vi "20 Log To File.vi"() -> ()   [LabVIEW 2014]
uses:
  <userlib>/_OpenG.lib/file/file.llb/Build Path - Traditional__ogtk.vi
  <vilib>/NI/LogRotate/LogRotate.lvclass
  Sensor Reading.ctl
  <vilib>/NI/LogRotate/options.ctl
panel:
  in  "Options":T1={"max file size (bytes)"=25000, "rotate count"=5, "max age (days)"=-1.0, "No archive dir"=TRUE, "Archive dir"=path ""}
  in  "Database File":path=path "C:/developer/New Model/database.txt"
  in  "Message Q":refnum<queue>
  in  "Data Q":refnum<queue>
  in  "Sensor Reading":T2
  # "INPUT PARAMETERS"
  # "INTERNAL VARIABLES - could possibly be set programatically..."
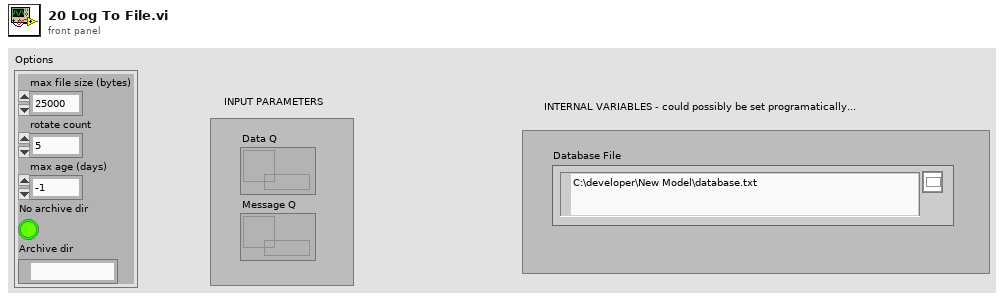
[diagram p1: front panel]
types:
  T1 = typedef "LogRotate.lvclass/options.ctl" = cluster{"max file size (bytes)":i64, "rotate count":u32, "max age (days)":dbl, "No archive dir":bool, "Archive dir":path}
  T2 = typedef "Sensor Reading.ctl" = cluster{"Sensor Name":string, "Timestamp":string, "Data Chunk":string}
  T3 = enum16{"open", "replace", "create", "open or create", "replace or create", "replace or create with confirmation"}
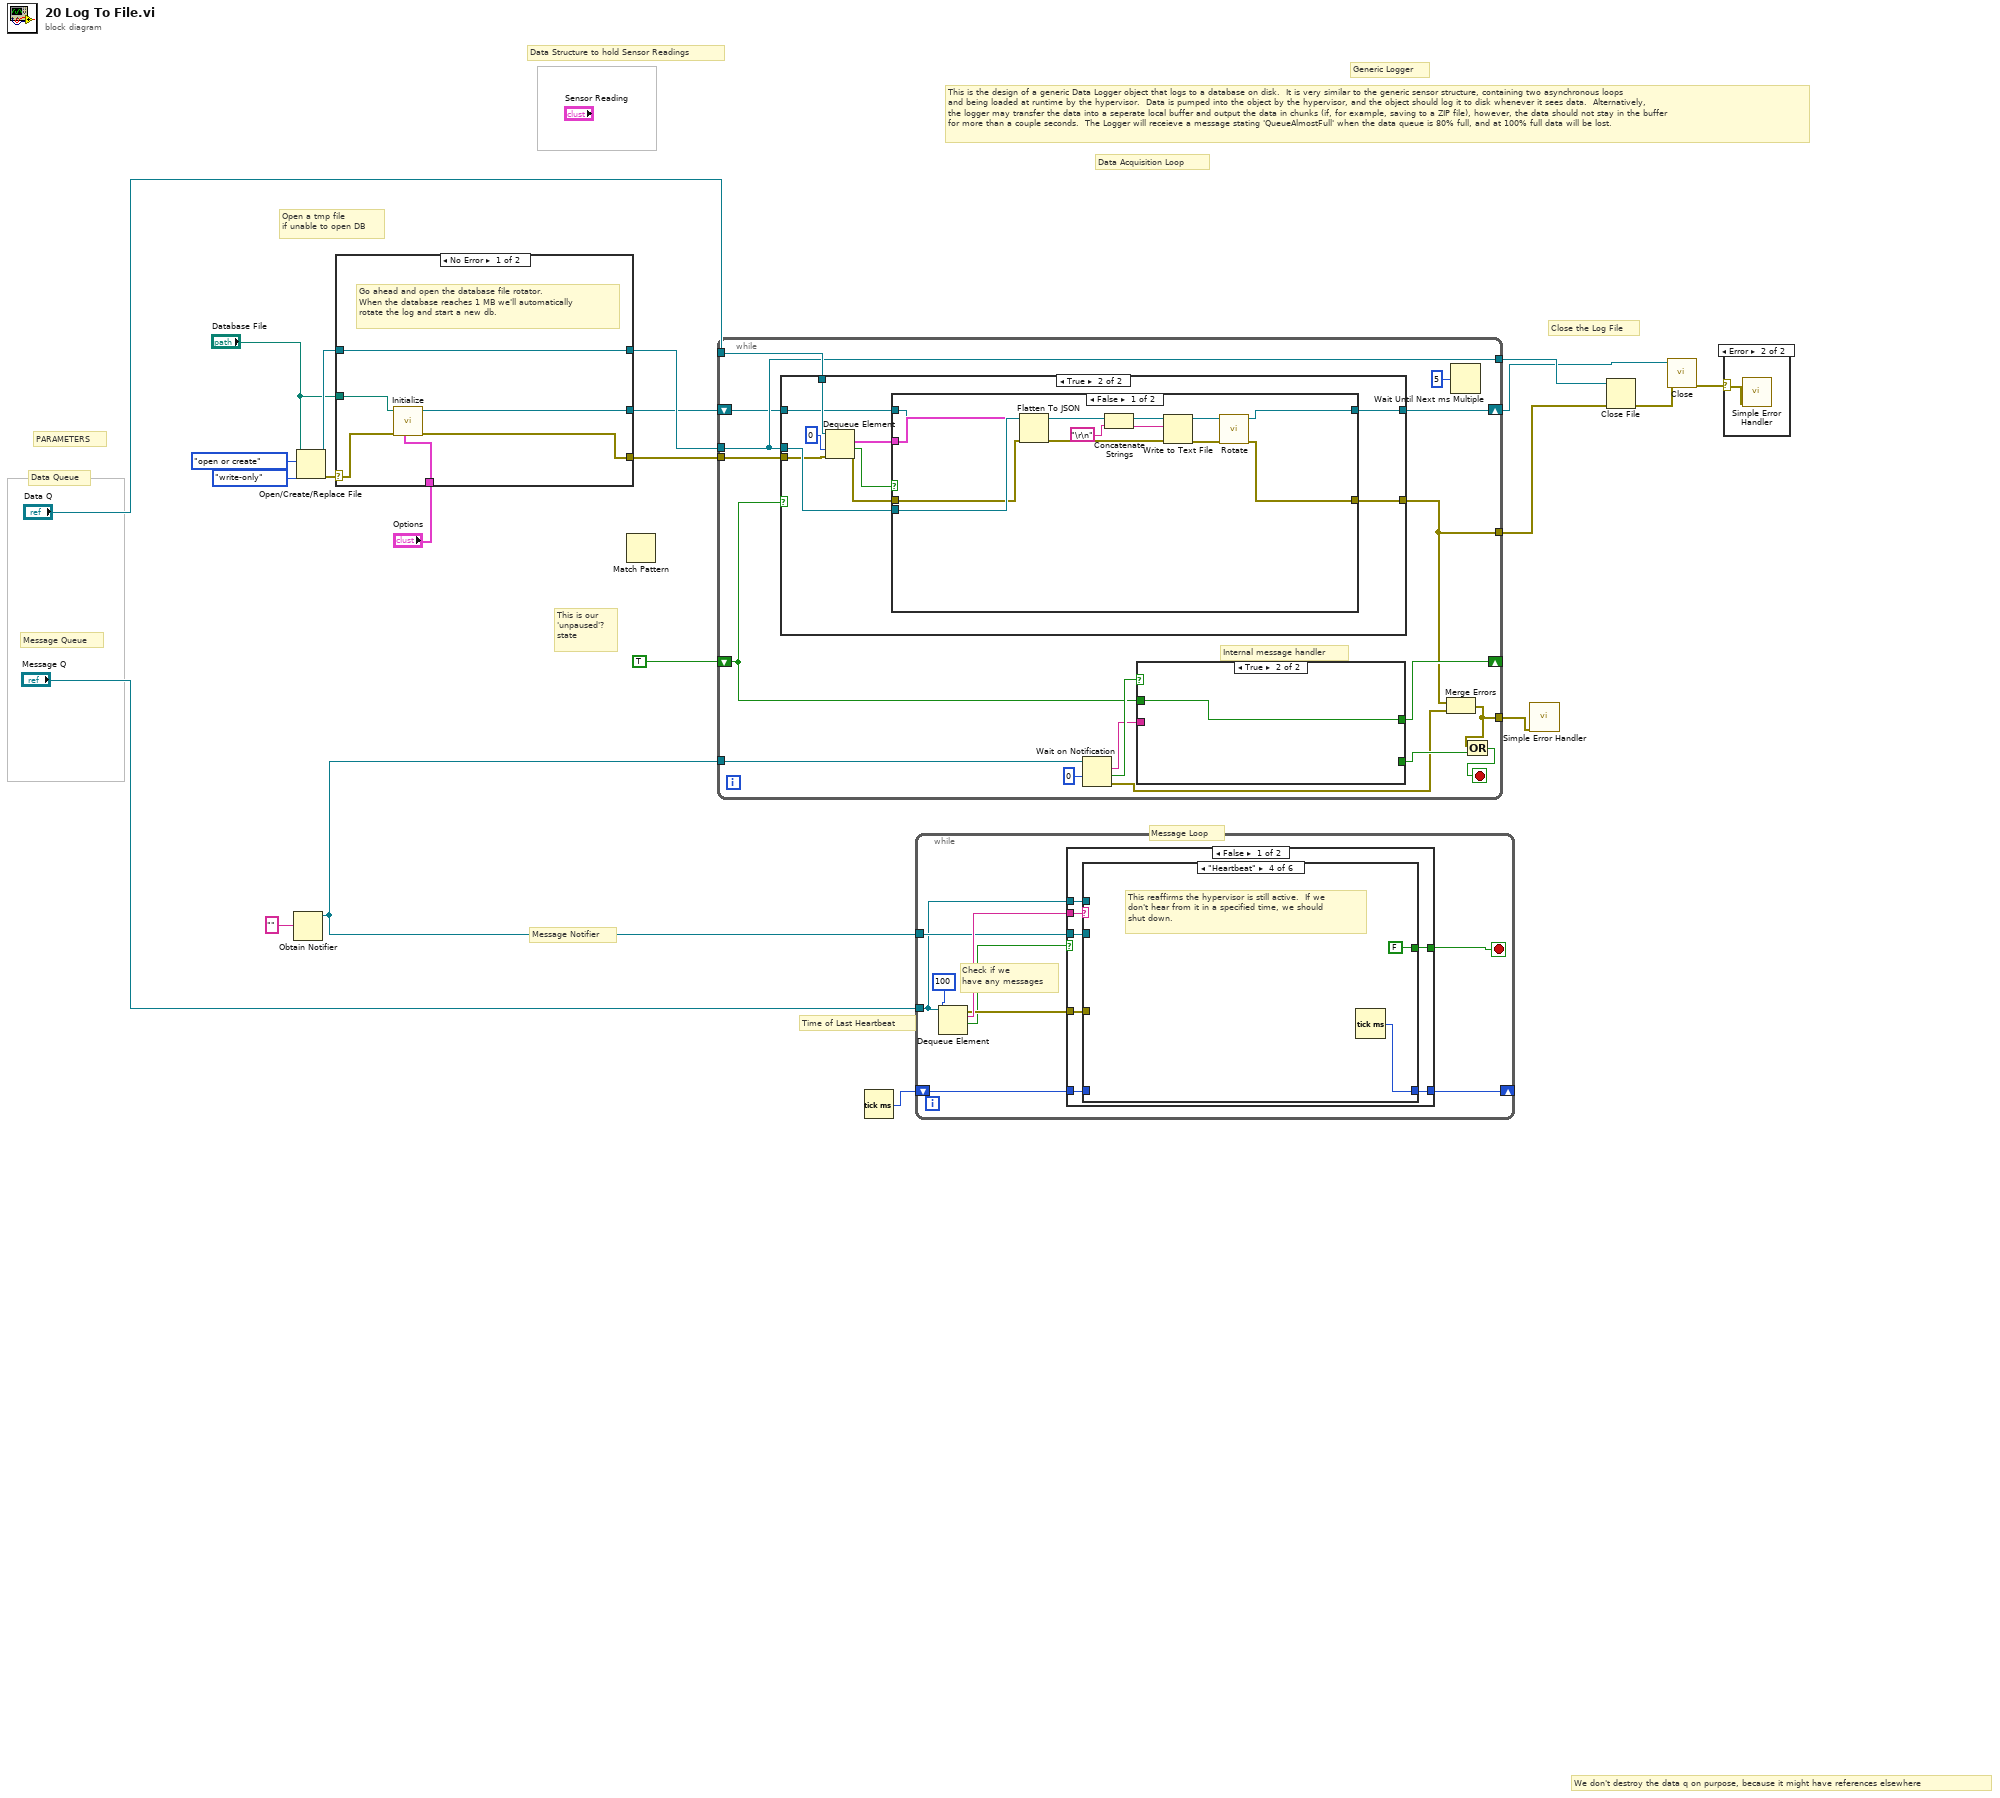
[diagram p0: block diagram]
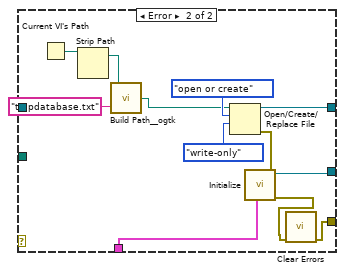
[diagram p3: hidden frame]
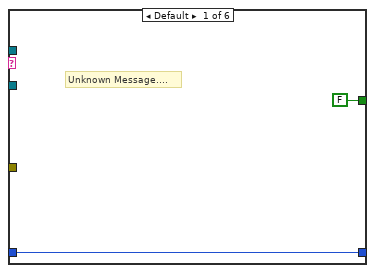
[diagram p4: hidden frame]
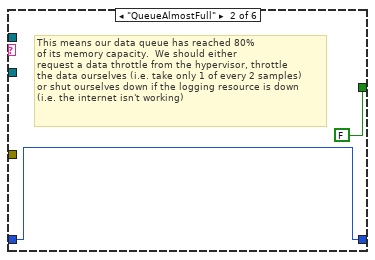
[diagram p5: hidden frame]
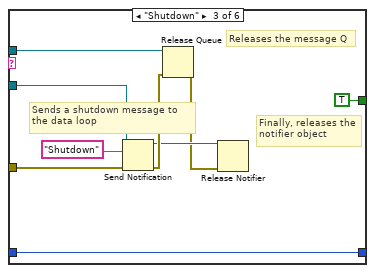
[diagram p6: hidden frame]
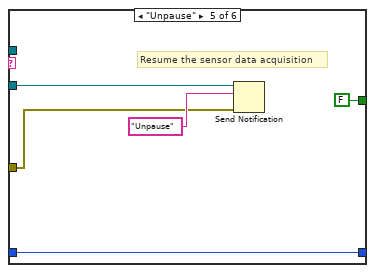
[diagram p7: hidden frame]
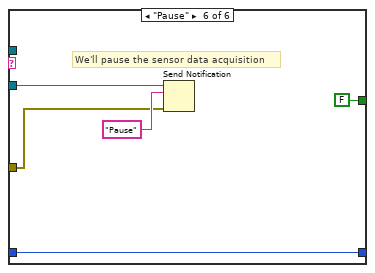
[diagram p8: hidden frame]
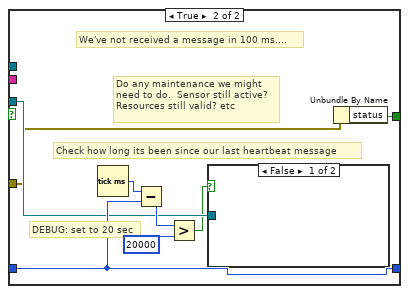
[diagram p9: hidden frame]
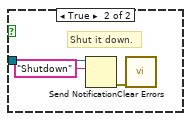
[diagram p10: hidden frame]
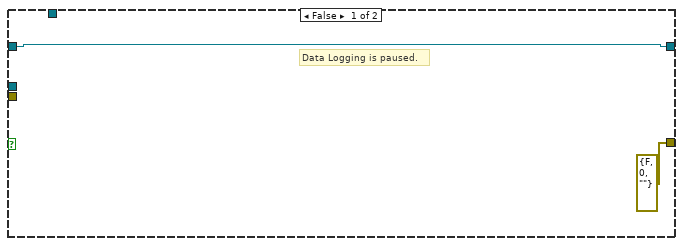
[diagram p11: hidden frame]
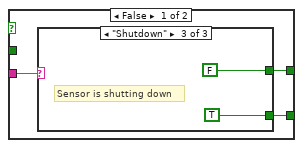
[diagram p13: hidden frame]
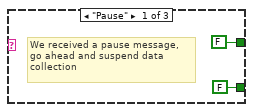
[diagram p14: hidden frame]
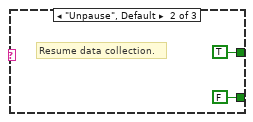
[diagram p15: hidden frame]
diagram:
  # "Time of Last Heartbeat"
  # "Close the Log File"
  # "Open a tmp file\nif unable to open DB"
  # "This is the design of a generic Data Logger object that logs to a database on disk.  It is very similar to the generic sensor structure, containing two asynchronous loops\nand being loaded at runtime by the hypervisor.  Data is pumped into the object by the hypervisor, and the object should log it to disk whenever it sees data.  Alternatively,\nthe logger may transfer the data into a seperate local buffer and output the data in chunks (if, for example, saving to a ZIP file), however, the data should not stay in the buffer\nfor more than a couple seconds.  The Logger will receieve a message stating 'QueueAlmostFull' when the data queue is 80% full, and at 100% full data will be lost."
  # "This is our\n'unpaused'?\nstate"
  # "We don't destroy the data q on purpose, because it might have references elsewhere"
  # "Data Structure to hold Sensor Readings"
  # "Data Acquisition Loop"
  # "Message Loop"
  # "Message Notifier"
  # "Message Queue"
  # "Data Queue"
  # "PARAMETERS"
  # "Generic Logger"
  n1 = Obtain Notifier(notification data type="") -> (notifier out=w21:refnum<notifier>)  [unwired: 3 in, 2 out]
  n2 = Open/Create/Replace File(file path (use dialog)="Database File", operation (0:open)=T3."open or create", access (0:read/write)=enum16{"read/write", "read-only", "write-only"}."write-only") -> (refnum out=w15:refnum<file>, error out=w16:errorcluster)  [unwired: 3 in, 1 out]
  n3 = case shown="No Error" w16 {
    selector: w16 -> [w25 _]
    tunnel: w15 -> [w27 _]
    tunnel: [w27 w29] -> w14
    tunnel: "Database File" -> [w26 _]
    tunnel: [w24 w33] -> w7
    tunnel: "Options" -> [w23 w30]
    tunnel: [w22 w28] -> w2
    frame No Error {
      # "Go ahead and open the database file rotator.\nWhen the database reaches 1 MB we'll automatically\nrotate the log and start a new db."
      n4 = call <vilib>:"Initialize.vi"("Options"=w23, "error in (no error)"=w25, "Log File Path"=w26) -> ("error out"=w22:errorcluster, "LogRotate"=w24:refnum<class "LogRotate.lvclass">)  [unwired: 7 in]
    }
    frame Error {
      n5 = Current VI's Path() -> (path=w35:path)
      n6 = Strip Path(path=w35) -> (stripped path=w34:path)  [unwired: 1 out]
      n7 = call-poly <userlib>:"Build Path__ogtk.vi"("name or relative path"="tmpdatabase.txt", "base path"=w34) -> ("appended path"=w36:path)
      n8 = Open/Create/Replace File(file path (use dialog)=w36, operation (0:open)=T3."open or create", access (0:read/write)=enum16{"read/write", "read-only", "write-only"}."write-only") -> (refnum out=w29:refnum<file>, error out=w32:errorcluster)  [unwired: 3 in, 1 out]
      n9 = call <vilib>:"Initialize.vi"("Options"=w30, "error in (no error)"=w32) -> ("error out"=w31:errorcluster, "LogRotate"=w33:refnum<class "LogRotate.lvclass">)  [unwired: 8 in]
      n10 = call <vilib>:"Clear Errors.vi"("error in (no error)"=w31) -> ("error out"=w28:errorcluster)  [unwired: 5 in, 1 out]
    }
  }
  n11 = Match Pattern() -> ()  [unwired: 3 in, 4 out]
  n12 = while {
    tunnel: "Data Q" -> [w47]
    tunnel: w21 -> [w56]
    shift-right: [w52] -> _
    shift-left: TRUE -> [w51]
    tunnel: w14 -> [w46]
    tunnel: [w46] -> w13
    tunnel: [w45] -> w12
    shift-right: [w42] -> w1
    shift-left: w7 -> [w43]
    tunnel: [w41] -> w3
    tunnel: w2 -> [w40]
    stop <- w49 stop-if-true
    # "Internal message handler"
    n13 = case shown="True" w51 {
      tunnel: w47 -> [_ w68]
      tunnel: w46 -> [_ w64]
      tunnel: [errorcluster {"status"=FALSE, "code"=0, "source"=""} ("error out") w63] -> w45
      tunnel: w43 -> [w57 w61]
      tunnel: [w57 w60] -> w42
      tunnel: w40 -> [_ w59]
      frame False {
        # "Data Logging is paused."
      }
      frame True {
        n14 = Dequeue Element(queue=w68, timeout in ms (-1)=0, error in (no error)=w59) -> (element=w65:T2, timed out?=w66:bool, error out=w62:errorcluster)  [unwired: 1 out]
        n15 = case shown="False" w66 {
          tunnel: w65 -> [w78 _]
          tunnel: w64 -> [w79 _]
          tunnel: [w74 w81] -> w63
          tunnel: w62 -> [w76 w81]
          tunnel: w61 -> [w77 w80]
          tunnel: [w69 w80] -> w60
          frame False {
            n16 = Flatten To JSON(anything=w78, error in (no error)=w76) -> (JSON string=w72:string, 11:w75:errorcluster)  [unwired: 1 in]
            n17 = Concatenate Strings(w72, "\r\n") -> (w70:string)
            n18 = Write to Text File(file (use dialog)=w79, text=w70, error in=w75) -> (error out=w73:errorcluster)  [unwired: 1 in, 2 out]
            n19 = call <vilib>:"Rotate.vi"("error in (no error)"=w73, "LogRotate in"=w77) -> ("error out"=w74:errorcluster, "LogRotate out"=w69:refnum<class "LogRotate.lvclass">)  [unwired: 8 in]
          }
          frame True {
          }
        }
      }
    }
    n20 = Wait on Notification(notifier=w56, timeout in ms (-1)=0) -> (notification=w53:string, timed out?=w54:bool, error out=w44:errorcluster)  [unwired: 2 in, 1 out]
    n21 = case shown="True" w54 {
      tunnel: w53 -> [w84 _]
      tunnel: [w83 _] -> w50
      tunnel: [w82 w91] -> w52
      tunnel: w51 -> [_ w91]
      frame False {
        n22 = case shown="\"Shutdown\"" w84 {
          tunnel: [FALSE FALSE TRUE] -> w83
          tunnel: [FALSE TRUE FALSE] -> w82
          frame "Pause" {
            # "We received a pause message,\ngo ahead and suspend data collection"
          }
          frame "Unpause", Default {
            # "Resume data collection."
          }
          frame "Shutdown" {
            # "Sensor is shutting down"
          }
        }
      }
      frame True {
      }
    }
    n23 = Merge Errors(w45, w44) -> (w41:errorcluster)
    n24 = Wait Until Next ms Multiple(millisecond multiple=u32 5) -> ()  [unwired: 1 out]
    n25 = Or(x=w41, y=w50) -> (x .or. y?=w49:bool)
  }
  n26 = Tick Count (ms)() -> (millisecond timer value=w9:u32)
  n27 = while {
    tunnel: "Message Q" -> [w97]
    tunnel: w21 -> [w98]
    shift-right: [w92] -> _
    shift-left: w9 -> [w93]
    stop <- w99 stop-if-true
    # "Check if we \nhave any messages"
    n28 = Dequeue Element(queue=w97, timeout in ms (-1)=100) -> (element=w100:string, timed out?=w94:bool, error out=w96:errorcluster)  [unwired: 1 in, 1 out]
    n29 = case shown="False" w94 {
      tunnel: w100 -> [w107 _]
      tunnel: [w106 w133] -> w99
      tunnel: w98 -> [w105 w136]
      tunnel: w97 -> [w104 _]
      tunnel: w96 -> [w103 w134]
      tunnel: w93 -> [w102 w137]
      tunnel: [w101 w137] -> w92
      frame False {
        n30 = case shown="\"Heartbeat\"" w107 {
          tunnel: [FALSE FALSE TRUE FALSE FALSE FALSE] -> w106
          tunnel: w105 -> [_ _ w118 _ w125 w129]
          tunnel: w104 -> [_ _ w119 _ _ _]
          tunnel: w103 -> [_ _ w117 _ w126 w130]
          tunnel: w102 -> [w108 w110 w112 _ w123 w128]
          tunnel: [w108 w110 w112 w122 w123 w128] -> w101
          frame Default {
            # "Unknown Message...."
          }
          frame "QueueAlmostFull" {
            # "This means our data queue has reached 80%\nof its memory capacity.  We should either\nrequest a data throttle from the hypervisor, throttle\nthe data ourselves (i.e. take only 1 of every 2 samples)\nor shut ourselves down if the logging resource is down\n(i.e. the internet isn't working)"
          }
          frame "Shutdown" {
            # "Finally, releases the\nnotifier object"
            # "Releases the message Q"
            # "Sends a shutdown message to \nthe data loop"
            n31 = Send Notification(notification="Shutdown", notifier=w118, error in (no error)=w117) -> (notifier out=w114:refnum<notifier>, error out=w116:errorcluster)
            n32 = Release Queue(queue=w119, error in (no error)=w116) -> (error out=w113:errorcluster)  [unwired: 1 in, 2 out]
            n33 = Release Notifier(notifier=w114, error in (no error)=w113) -> ()  [unwired: 1 in, 3 out]
          }
          frame "Heartbeat" {
            # "This reaffirms the hypervisor is still active.  If we\ndon't hear from it in a specified time, we should\nshut down."
            n34 = Tick Count (ms)() -> (millisecond timer value=w122:u32)
          }
          frame "Unpause" {
            # "Resume the sensor data acquisition"
            n35 = Send Notification(notification="Unpause", notifier=w125, error in (no error)=w126) -> ()  [unwired: 2 out]
          }
          frame "Pause" {
            # "We'll pause the sensor data acquisition"
            n36 = Send Notification(notification="Pause", notifier=w129, error in (no error)=w130) -> ()  [unwired: 2 out]
          }
        }
      }
      frame True {
        # "DEBUG: set to 20 sec"
        # "Check how long its been since our last heartbeat message"
        # "Do any maintenance we might\nneed to do.  Sensor still active?\nResources still valid? etc"
        # "We've not received a message in 100 ms...."
        n37 = Tick Count (ms)() -> (millisecond timer value=w140:u32)
        n38 = Subtract(x=w140, y=w137) -> (x-y=w139:u32)
        n39 = Greater?(x=w139, y=u32 20000) -> (0:w135:bool)
        n40 = case shown="False" w135 {
          tunnel: w136 -> [_ w143]
          frame False {
          }
          frame True {
            # "Shut it down."
            n41 = Send Notification(notification="Shutdown", notifier=w143) -> (error out=w141:errorcluster)  [unwired: 1 in, 1 out]
            n42 = call <vilib>:"Clear Errors.vi"("error in (no error)"=w141) -> ()  [unwired: 5 in, 2 out]
          }
        }
        n43 = Unbundle By Name(w134) -> ("status"=w133:bool)
      }
    }
  }
  n44 = call <vilib>:"Simple Error Handler.vi"("error in (no error)"=w3) -> ()  [unwired: 4 in, 5 out]
  n45 = Close File(refnum=w13, error in=w12) -> (error out=w5:errorcluster)  [unwired: 1 out]
  n46 = call <vilib>:"Close.vi"("error in (no error)"=w5, "LogRotate"=w1) -> ("error out"=w4:errorcluster)  [unwired: 9 in]
  n47 = case shown="Error" w4 {
    selector: w4 -> [_ w144]
    frame No Error {
    }
    frame Error {
      n48 = call <vilib>:"Simple Error Handler.vi"("error in (no error)"=w144) -> ()  [unwired: 4 in, 5 out]
    }
  }
